vi "Test MQTT-4.7.2-1.vi"(8 "error in (no error)":errorcluster) -> (0 "error out":errorcluster)   [LabVIEW 2013]
uses:
  <vilib>/addons/_JKI Toolkits/Caraya/classes/Test/Test.lvclass
  source/TopicFilter/_TopicFilter.lvclass
  <vilib>/addons/_JKI Toolkits/Caraya/classes/Assert/Assert.lvclass
panel:
  out "Match":bool
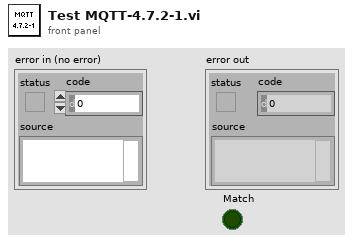
[diagram p1: front panel]
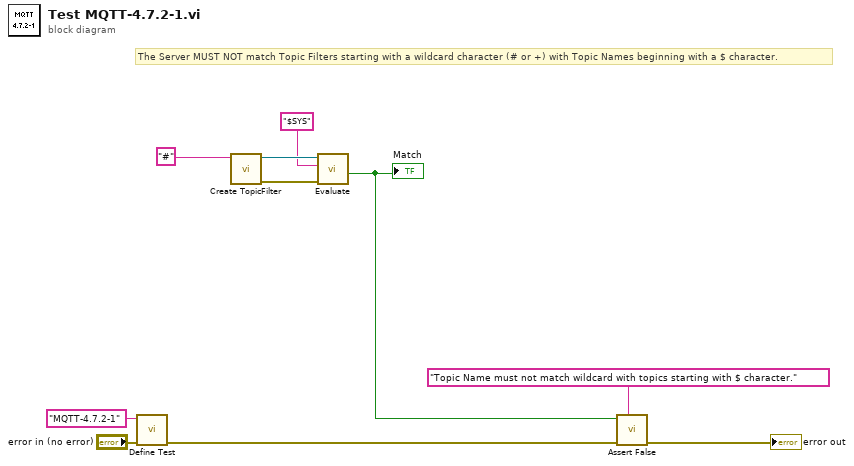
[diagram p0: block diagram]
diagram:
  # "The Server MUST NOT match Topic Filters starting with a wildcard character (# or +) with Topic Names beginning with a $ character."
  n1 = call <vilib>:"Define Test.vi"("error in (no error)"="error in (no error)", "Label (VI Title)"="MQTT-4.7.2-1") -> ("error out"=w7:errorcluster)  [unwired: 9 in]
  n2 = call "Create TopicFilter.vi"("Topic Filter"="#" ("Topic")) -> ("error out"=w5:errorcluster, "TopicFilter out"=w4:refnum<class "_TopicFilter.lvclass">)  [unwired: 9 in]
  n3 = call "Evaluate.vi"("error in (no error)"=w5, "Topic"="$SYS" ("Topic Filter"), "TopicFilter in"=w4) -> ("Match"=w3:bool)  [unwired: 5 in, 3 out]
  "Match" <- w3
  n4 = call <vilib>:"Assert False.vi"("Label"="Topic Name must not match wildcard with topics starting with $ character.", "error in (no error)"=w7, "False?"=w3) -> ("error out"=→"error out":errorcluster)  [unwired: 8 in]
